vi "CheckLoadLib.vi"(0 "Host_Reference":refnum<class "HGF_Reference.lvclass">, 2 "timeout in ms (-1)":i32=-1, 3 "LibraryName":string, 4 "classname":string, 5 "error in (no error)":errorcluster) -> (14 "dup Host_Reference":refnum<class "HGF_Reference.lvclass">, 16 "status":bool)   [LabVIEW 2009, in "MoAgSy.lvlib" / "MoAgSy_Host.lvclass"]
uses:
  MoAgSy_Host.lvclass
  HGF_BaseClasses/HGF_Reference/HGF_Reference.lvclass
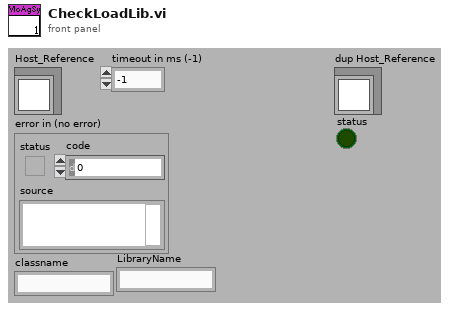
[diagram p1: front panel]
types:
  T1 = cluster{"Working Folder":path, "Class Folder":path}
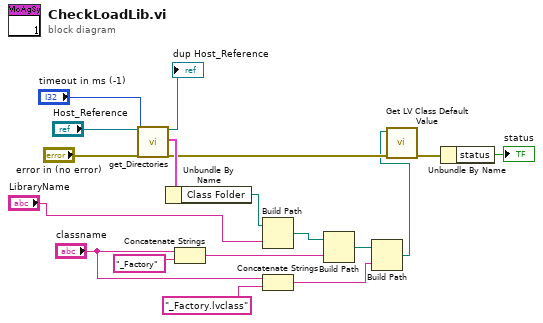
[diagram p0: block diagram]
diagram:
  n1 = call "get_Directories.vi"("Host_Reference"="Host_Reference", "timeout in ms (-1)"="timeout in ms (-1)", "error in (no error)"="error in (no error)") -> ("dup Host_Reference"=→"dup Host_Reference":refnum<class "HGF_Reference.lvclass">, "Directories"=w14:T1, "error out"=w13:errorcluster)  [unwired: 14 in]
  n2 = Unbundle By Name(w14) -> ("Class Folder"=w12:path)
  n3 = Concatenate Strings("classname", "_Factory" ("string")) -> (w3:string)
  n4 = Build Path(base path=w12, name or relative path="LibraryName") -> (appended path=w11:path)
  n5 = Concatenate Strings("classname", "_Factory.lvclass" ("string")) -> (w1:string)
  n6 = Build Path(base path=w11, name or relative path=w3) -> (appended path=w5:path)
  n7 = Build Path(base path=w5, name or relative path=w1) -> (appended path=w6:path)
  n8 = call <vilib>:"Get LV Class Default Value.vi"("error in (no error)"=w13, "class path"=w6) -> ("error out"=w9:errorcluster)  [unwired: 8 in, 1 out]
  n9 = Unbundle By Name(w9) -> ("status"=→"status":bool)
